vi "WriteReport.vi"(8 "error in (no error)":errorcluster, 9 "StepName":string, 10 "Pass/Fail":bool, 11 "输出簇":T1) -> (0 "error out":errorcluster caption="error out (no error)", 1 "DBresult":bool)   [LabVIEW 2013]
uses:
  GlobValue.vi
  <vilib>/Utility/file.llb/Write To Spreadsheet File (string).vi
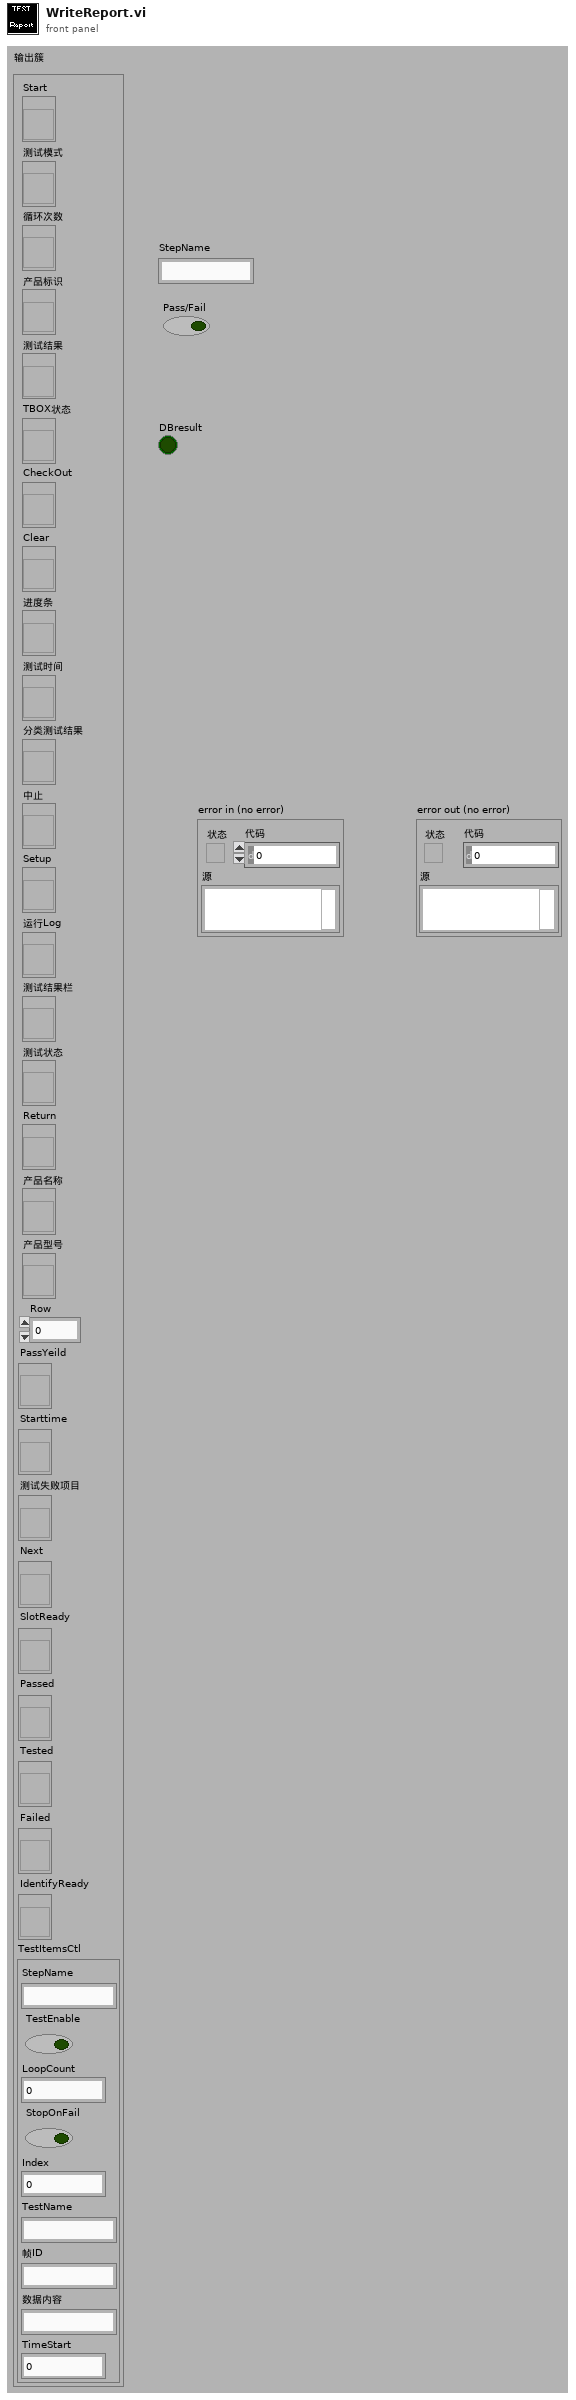
[diagram p1: front panel]
types:
  T1 = typedef "控件.ctl" = cluster{"Start":refnum<vi>, "测试模式":refnum<vi>, "循环次数":refnum<vi>, "产品标识":refnum<vi>, "测试结果":refnum<vi>, "TBOX状态":refnum<vi>, "CheckOut":refnum<vi>, "Clear":refnum<vi>, "进度条":refnum<vi>, "测试时间":refnum<vi>, "分类测试结果":refnum<vi>, "中止":refnum<vi>, "Setup":refnum<vi>, "运行Log":refnum<vi>, "测试结果栏":refnum<vi>, "测试状态":refnum<vi>, "Return":refnum<vi>, "产品名称":refnum<vi>, "产品型号":refnum<vi>, "Row":i32, "PassYeild":refnum<vi>, "Starttime":refnum<vi>, "测试失败项目":refnum<vi>, "Next":refnum<vi>, "SlotReady":refnum<vi>, "Passed":refnum<vi>, "Tested":refnum<vi>, "Failed":refnum<vi>, "IdentifyReady":refnum<vi>, "TestItemsCtl":cluster{"StepName":string, "TestEnable":bool, "LoopCount":u32, "StopOnFail":bool, "Index":u32, "TestName":string, "帧ID":string, "数据内容":string, "TimeStart":u32}}
  T2 = enum16{"open", "replace", "create", "open or create", "replace or create", "replace or create with confirmation"}
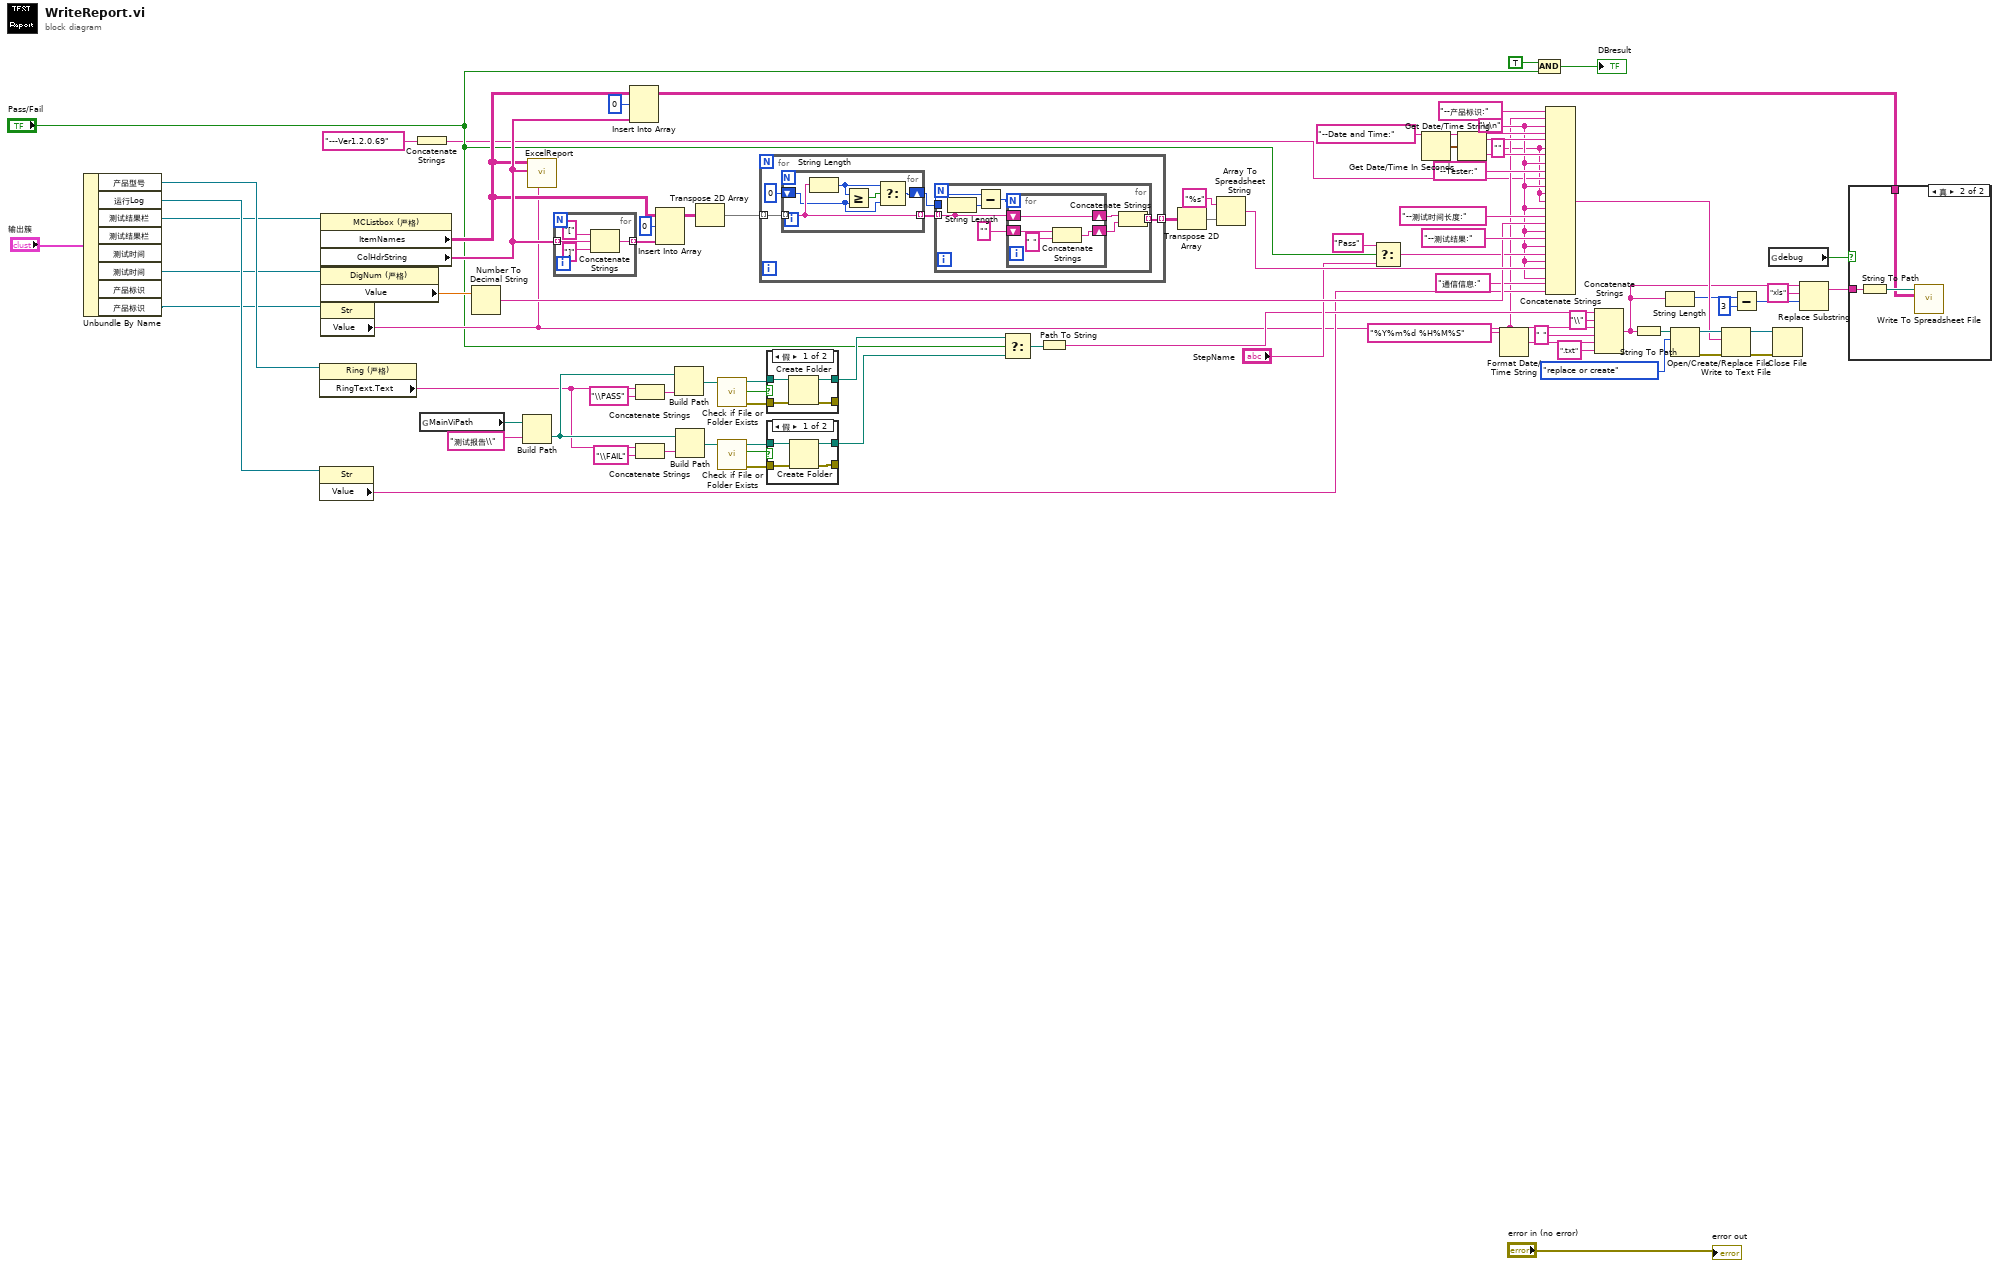
[diagram p0: block diagram]
diagram:
  w4 = "" ("字符串")
  w36 = "\r\n"
  n1 = Unbundle By Name("输出簇") -> ("产品型号"=w28:refnum<vi>, "运行Log"=w32:refnum<vi>, "测试结果栏"=w1:refnum<vi>, "测试时间"=w2:refnum<vi>, "产品标识"=w3:refnum<vi>)  [unwired: 3 out]
  n2 = property class="Ring (严格)"(reference=w28) -> ("RingText.Text"=w5:string)  [unwired: 1 in, 2 out]
  n3 = property class="Str"(reference=w32) -> ("Value"=w31:string)  [unwired: 1 in, 2 out]
  n4 = property class="MCListbox (严格)"(reference=w1) -> ("ItemNames"=w13:string[][], "ColHdrString"=w17:string[])  [unwired: 1 in, 2 out]
  n5 = property class="DigNum (严格)"(reference=w2) -> ("Value"=w53:dbl)  [unwired: 1 in, 2 out]
  n6 = property class="Str"(reference=w3) -> ("Value"=w12:string)  [unwired: 1 in, 2 out]
  n7 = Concatenate Strings("---Ver1.2.0.69" ("字符串")) -> (w8:string)
  n8 = global read "GlobValue.vi" "MainViPath"() -> (w30:path)
  n9 = Number To Decimal String(number=w53) -> (decimal integer string=w55:string)  [unwired: 1 out]
  n10 = Build Path(base path=w30, name or relative path="测试报告\\" ("名称或相对路径")) -> (appended path=w29:path)
  n11 = call "ExcelReport.vi"("SN"=w12, "列首字符串"=w17, "TestResults"=w13) -> ()  [unwired: 8 in, 1 out]
  n12 = for "For循环" {
    tunnel: w17 -> [w84] mode=indexing
    tunnel: [w82] -> w69 mode=indexing
    n13 = Concatenate Strings("[" ("字符串"), w84, "]" ("字符串")) -> (w82:string)
  }
  n14 = Insert Into Array(array=w13, index (row)=0 ("索引 (行)"), new element=w17) -> (w15:string[][])  [unwired: 1 in]
  n15 = Concatenate Strings(w5, "\\PASS" ("name or relative path")) -> (w27:string)
  n16 = Concatenate Strings(w5, "\\FAIL" ("name or relative path")) -> (w24:string)
  n17 = Insert Into Array(array=w13, index (row)=0 ("索引 (行)"), new element=w69) -> (w72:string[][])  [unwired: 1 in]
  n18 = Build Path(base path=w29, name or relative path=w27) -> (appended path=w48:path)
  n19 = Build Path(base path=w29, name or relative path=w24) -> (appended path=w47:path)
  n20 = Transpose 2D Array(2D array=w72) -> (transposed array=w80:string[][])
  n21 = call <vilib>:"Check if File or Folder Exists.vi"("path"=w48) -> ("error out"=w52:errorcluster, "file or folder exists?"=w39:bool, "dup path"=w51:path)  [unwired: 1 in, 7 out]
  n22 = call <vilib>:"Check if File or Folder Exists.vi"("path"=w47) -> ("error out"=w49:errorcluster, "file or folder exists?"=w38:bool, "dup path"=w50:path)  [unwired: 1 in, 7 out]
  n23 = for "For循环" {
    tunnel: w80 -> [w88] mode=indexing
    tunnel: [w87] -> w79 mode=indexing
    n24 = for "For循环" {
      tunnel: w88 -> [w107] mode=indexing
      shift-right: [w103] -> w86
      shift-left: 0 -> [w105]
      tunnel: [w107] -> w89 mode=indexing
      n25 = String Length(string=w107) -> (length=w106:i32)
      n26 = Greater Or Equal?(x=w106, y=w105) -> (x >= y?=w104:bool)
      n27 = Select(t=w106, s=w104, f=w105) -> (s? t:f=w103:i32)
    }
    n28 = for "For循环" {
      tunnel: w89 -> [w91] mode=indexing
      tunnel: [w96] -> w87 mode=indexing
      tunnel: w86 -> [w94]
      n29 = String Length(string=w91) -> (length=w98:i32)
      n30 = Subtract(x=w94, y=w98) -> (x-y=w97:i32)
      n31 = for "For循环" {
        N: w97 -> [_]
        shift-right: [w100] -> w93
        shift-left: "" -> [w101]
        shift-right: [w99] -> w92
        shift-left: w91 -> [w99]
        n32 = Concatenate Strings(w101, " ") -> (w100:string)
      }
      n33 = Concatenate Strings(w92, w93) -> (w96:string)
    }
  }
  n34 = case shown="假" w39 {
    tunnel: w51 -> [w111 w112]
    tunnel: [w110 _] -> _
    tunnel: w52 -> [w109 _]
    tunnel: [w108 w112] -> w43
    frame False {
      n35 = Create Folder(path (use dialog)=w111, error in=w109) -> (created path=w108:path, error out=w110:errorcluster)  [unwired: 2 out]
    }
    frame True {
    }
  }
  n36 = case shown="假" w38 {
    tunnel: w50 -> [w116 w117]
    tunnel: [w115 _] -> _
    tunnel: w49 -> [w114 _]
    tunnel: [w113 w117] -> w42
    frame False {
      n37 = Create Folder(path (use dialog)=w116, error in=w114) -> (created path=w113:path, error out=w115:errorcluster)  [unwired: 2 out]
    }
    frame True {
    }
  }
  n38 = Select(t=w43, s="Pass/Fail", f=w42) -> (s? t:f=w41:path)
  n39 = Path To String(path=w41) -> (string=w40:string)
  n40 = Transpose 2D Array(2D array=w79) -> (transposed array=w73:string[][])
  n41 = Array To Spreadsheet String(array=w73, 3:"%s" ("format string")) -> (spreadsheet string=w76:string)  [unwired: 1 out]
  n42 = Select(t="Pass", s="Pass/Fail", f="StepName") -> (s? t:f=w44:string)
  n43 = Get Date/Time In Seconds() -> (seconds since 1Jan1904=w75:timestamp)
  n44 = Get Date/Time String(seconds (now)=w75) -> (date string=w60:string, time string=w59:string)  [unwired: 2 out]
  n45 = Format Date/Time String(time format string (%c)="%Y%m%d %H%M%S") -> (date/time string=w63:string)  [unwired: 2 out]
  n46 = And(x=TRUE, y="Pass/Fail") -> (x .and. y?=→"DBresult":bool)
  n47 = Concatenate Strings("--产品标识:" ("element"), w12, w36, "--Date and Time:" ("元素"), w60, w4, w59, w36, "--Tester:" ("element"), w8, w36, w4, w4, w36, "--测试时间长度:" ("字符串"), w55, w36, "--测试结果:" ("元素"), w36, w44, w36, w76, w36, "通信信息:" ("字符串"), w31) -> (w65:string)
  n48 = Concatenate Strings(w40, "\\" ("string"), w12, " " ("string"), w63, ".txt" ("字符串")) -> (w21:string)
  n49 = String To Path(string=w21) -> (path=w68:path)
  n50 = String Length(string=w21) -> (length=w23:i32)
  n51 = Open/Create/Replace File(file path (use dialog)=w68, operation (0:open)=T2."replace or create" ("操作(0:open)")) -> (refnum out=w67:refnum<file>, error out=w66:errorcluster)  [unwired: 1 in, 4 out]
  n52 = Write to Text File(file (use dialog)=w67, text=w65, error in=w66) -> (refnum out=w70:refnum<file>, error out=w71:errorcluster)  [unwired: 2 out]
  n53 = Subtract(x=w23, y=3) -> (x-y=w19:i32)
  n54 = global read "GlobValue.vi" "debug"() -> (w14:bool)
  n55 = Close File(refnum=w70, error in=w71) -> ()  [unwired: 2 out]
  n56 = Replace Substring(3:w19, 4:"xls" ("子字符串(\"\")"), 5:w21) -> (1:w18:string)  [unwired: 1 in, 1 out]
  n57 = case shown="真" w14 {
    tunnel: w18 -> [_ w120]
    tunnel: w15 -> [_ w118]
    frame False {
    }
    frame True {
      n58 = String To Path(string=w120) -> (path=w119:path)
      n59 = call-poly <vilib>:"Write To Spreadsheet File.vi"("2D data"=w118, "file path (dialog if empty)"=w119) -> ()  [unwired: 6 in, 1 out]
    }
  }
  "error out" <- "error in (no error)"
